vi "grab.vi"(4 "stop":bool, 8 "error in":errorcluster, 11 "Session In":T1) -> (0 "error out":errorcluster, 1 "Image Pixels (I16)":i16[][](array[numeric]), 2 "Image":T2(plugin-control), 3 "Session Out":T1)   [LabVIEW 2014]
uses:
  <vilib>/userdefined/High Color/IMAQdx.ctl
  <vilib>/vision/driver/NI_Vision_Acquisition_Software.lvlib
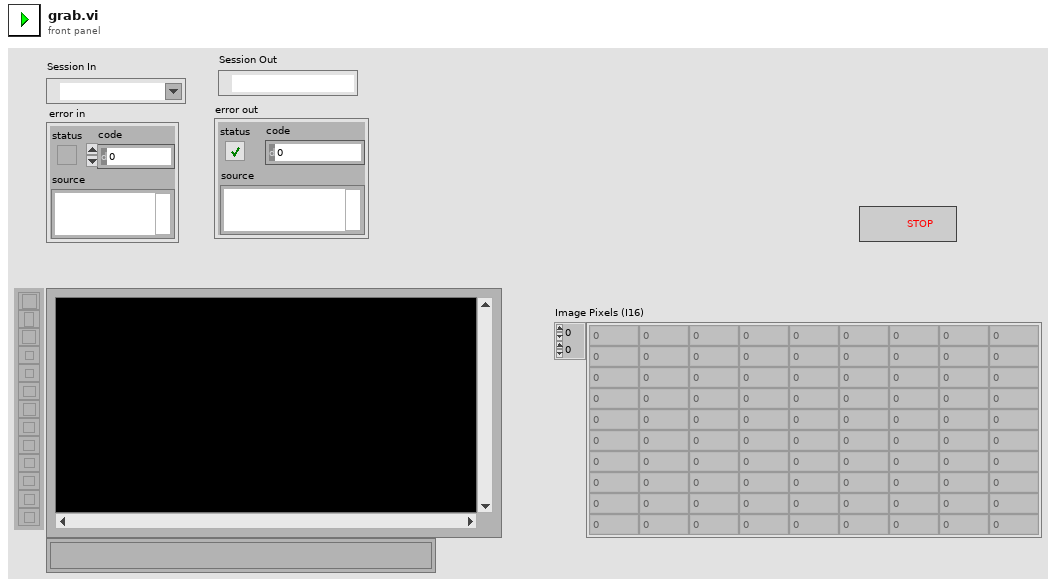
[diagram p1: front panel]
types:
  T1 = typedef "IMAQdx.ctl" = refnum<k21>
  T2 = typedef "IMAQ Image.ctl" = refnum<image>
  T3 = typedef "Image Type" = u32
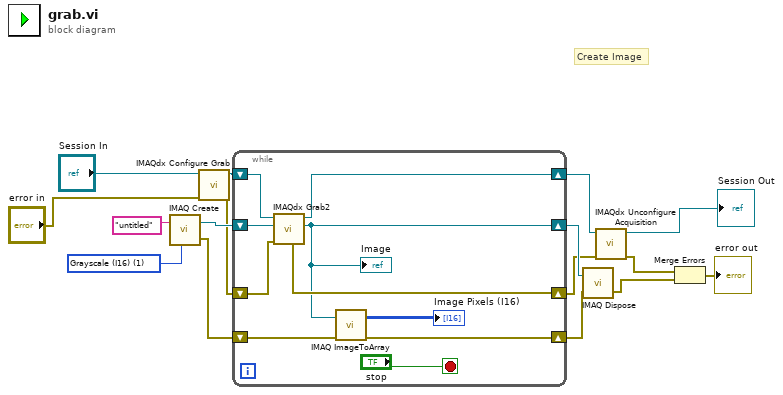
[diagram p0: block diagram]
diagram:
  w15 = T3 1 items=["Grayscale (U8)", "Grayscale (I16)", "Grayscale (SGL)", "Complex (CSG)", "RGB (U32)", "HSL (U32)", "RGB (U64)", "Grayscale (U16)"] ("Image Type")
  # "Create Image"
  n1 = call "IMAQ Create"("Image Name"="untitled", "Image Type"=w15) -> ("New Image"=w13:T2, "error out"=w7:errorcluster)  [unwired: 3 in]
  n2 = call <vilib>:"IMAQdx Configure Grab.vi"("error in"="error in", "Session In"="Session In") -> ("error out"=w12:errorcluster, "Session Out"=w16:T1)  [unwired: 8 in]
  n3 = while {
    shift-right: [w19] -> w11
    shift-left: w13 -> [w21]
    shift-right: [w24] -> w9
    shift-left: w16 -> [w25]
    shift-right: [w17] -> w6
    shift-left: w7 -> [w18]
    shift-right: [w22] -> w8
    shift-left: w12 -> [w23]
    stop <- "stop" stop-if-true
    n4 = call <vilib>:"IMAQdx Grab2.vi"("error in"=w23, "Image In"=w21, "Session In"=w25) -> ("error out"=w22:errorcluster, "Image Out"=w19:T2, "Session Out"=w24:T1)  [unwired: 5 in, 1 out]
    "Image" <- w19
    n5 = call "IMAQ ImageToArray"("error in (no error)"=w18, "Image"=w19) -> ("error out"=w17:errorcluster, "Image Pixels (I16)"=→"Image Pixels (I16)":i16[][])  [unwired: 2 in, 3 out]
  }
  n6 = call "IMAQ Dispose"("Image"=w11, "error in (no error)"=w6) -> ("error out"=w3:errorcluster)  [unwired: 4 in]
  n7 = call <vilib>:"IMAQdx Unconfigure Acquisition.vi"("error in"=w8, "Session In"=w9) -> ("error out"=w4:errorcluster, "Session Out"=→"Session Out":T1)  [unwired: 8 in]
  n8 = Merge Errors(w4, w3) -> (→"error out":errorcluster)
